vi "create extended nufern xmit string.vi"(8 "error in (no error)":errorcluster, 10 "Extended Operation":T1={"Extended Operation"=0, "OK Button"=FALSE, " HPE Photodiode \nSignal Drop Tolerance"=0.99} {"HPE Photodiode \nSignal Drop Tolerance" min=0.01 max=0.99 step=0.01 format="%#_g%%"; "Extended Operation" format="0x%x" items=["Set HPE Photodiode Signal Drop Tolerance"=67, "Get HPE Photodiode Signal Drop Tolerance"=68, "Switch HPE Photodiode Fault Enable"=69, "Get Temperature Sensor Status"=70, "Switch Communication Timeout Enable"=71]}, 11 "PAPA Address":i8=10 format="0x%02x") -> (0 "error out":errorcluster, 1 "String out":string, 2 "CRC Out":i32, 3 "String Out to nufern":string)   [LabVIEW 2016]
uses:
  Extended Operation Control 3.ctl
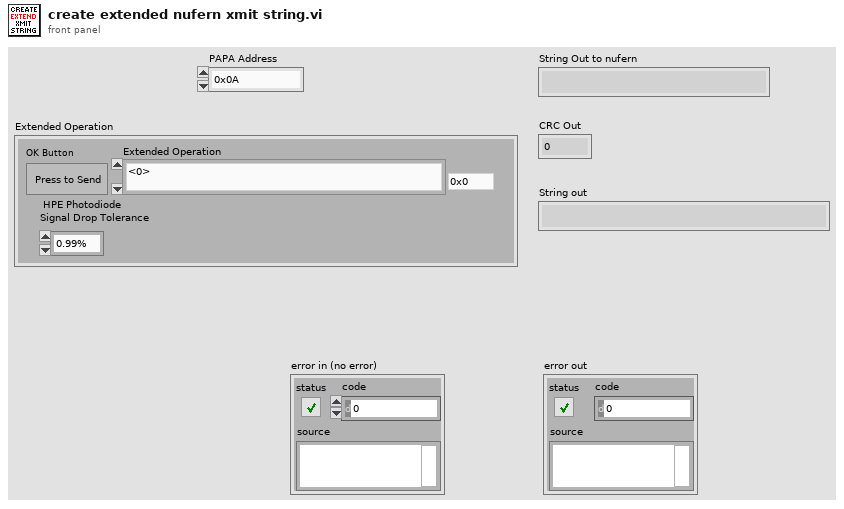
[diagram p1: front panel]
types:
  T1 = typedef "Extended Operation Control 3.ctl" = cluster{"Extended Operation":u16, "OK Button":bool, " HPE Photodiode \nSignal Drop Tolerance":dbl}
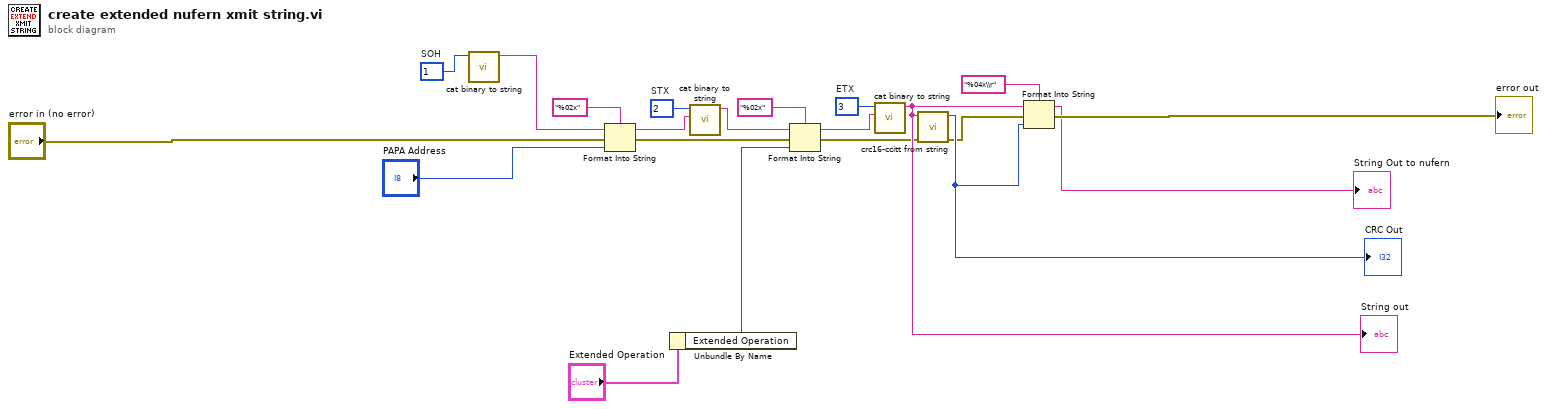
[diagram p0: block diagram]
diagram:
  w9 = 3  # ETX
  w16 = 2  # STX
  w18 = 1  # SOH
  n1 = call "cat binary to string.vi"("ETX"=w18) -> ("String out"=w19:string)  [unwired: 10 in]
  n2 = Format Into String(format string="%02x", initial string=w19, error in="error in (no error)", "PAPA Address") -> (resulting string=w15:string, error out=w13:errorcluster)
  n3 = Unbundle By Name("Extended Operation") -> ("Extended Operation"=w1:u16)
  n4 = call "cat binary to string.vi"("String in"=w15, "ETX"=w16) -> ("String out"=w17:string)  [unwired: 9 in]
  n5 = Format Into String(format string="%02x", initial string=w17, error in=w13, w1) -> (resulting string=w8:string, error out=w10:errorcluster)
  n6 = call "cat binary to string.vi"("String in"=w8, "ETX"=w9) -> ("String out"=w21:string)  [unwired: 9 in]
  "String out" <- w21
  n7 = call "crc16-ccitt from string.vi"("error in (no error)"=w10, "String"=w21) -> ("error out"=w11:errorcluster, "CRC Out"=w12:i32)  [unwired: 8 in]
  "CRC Out" <- w12
  n8 = Format Into String(format string="%04x\\r", initial string=w21, error in=w11, w12) -> (resulting string=→"String Out to nufern":string, error out=→"error out":errorcluster)
